vi "loadcontrsval.vi"(4 "error in":errorcluster, 5 "Array":refnum<vi>[](array[refnum]), 6 "Section":string, 7 "refnum in":T1) -> (0 "error out":errorcluster, 3 "refnum out":T1)   [LabVIEW 2010]
uses:
  <vilib>/Utility/config.llb/Config Data RefNum.ctl
  <vilib>/Utility/config.llb/Read Key (String).vi
  <vilib>/Utility/config.llb/Write Key (String).vi
  <vilib>/Utility/config.llb/Read Key (Path).vi
  <vilib>/Utility/config.llb/Write Key (Path).vi
  <vilib>/Utility/config.llb/Read Key (Double).vi
  <vilib>/Utility/config.llb/Write Key (Double).vi
  <vilib>/Utility/config.llb/Read Key (I32).vi
  <vilib>/Utility/config.llb/Write Key (I32).vi
  <vilib>/Utility/config.llb/Read Key (Boolean).vi
  <vilib>/Utility/config.llb/Write Key (Boolean).vi
  <vilib>/Utility/config.llb/NI_LVConfig.lvlib
panel:
  out "Array 2":string[](array[string])
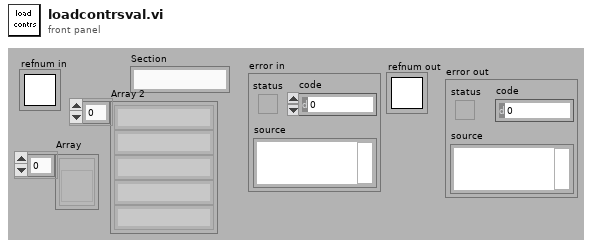
[diagram p1: front panel]
types:
  T1 = typedef "NI_LVConfig.lvlib/Config Data RefNum.ctl" = refnum<k1>
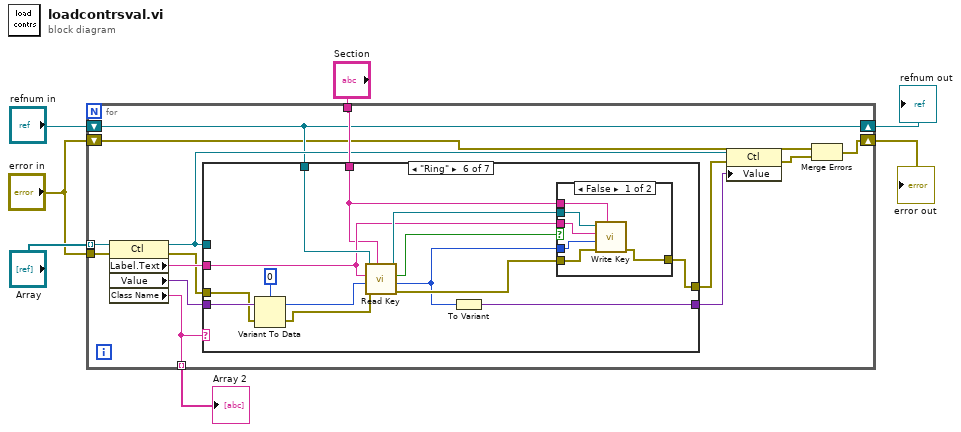
[diagram p0: block diagram]
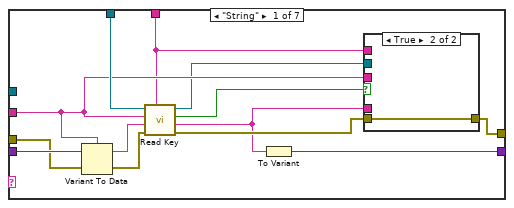
[diagram p2: hidden frame]
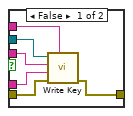
[diagram p3: hidden frame]
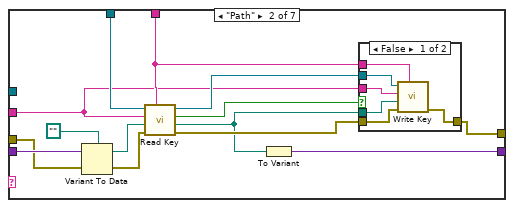
[diagram p4: hidden frame]
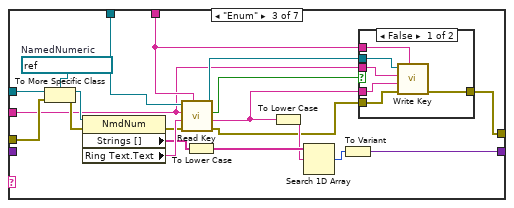
[diagram p6: hidden frame]
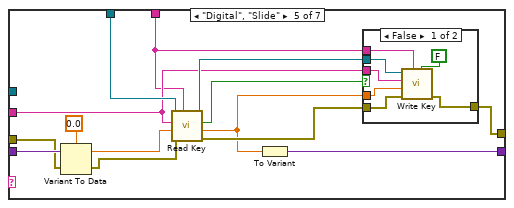
[diagram p9: hidden frame]
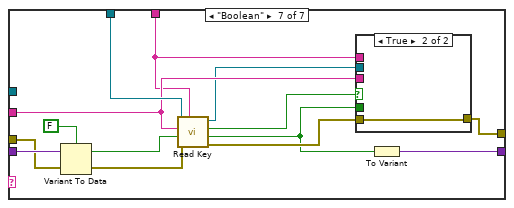
[diagram p12: hidden frame]
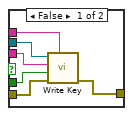
[diagram p13: hidden frame]
diagram:
  n1 = for {
    tunnel: "Section" -> [w18]
    tunnel: "Array" -> [w21] mode=indexing
    shift-right: [w14] -> w7
    shift-left: "refnum in" -> [w14]
    shift-right: [w9] -> w3
    shift-left: "error in" -> [w10]
    tunnel: [w20] -> w2 mode=indexing
    tunnel: "error in" -> [w11]
    n2 = property on="Property Node" class="Ctl"(reference=w21, error in=w11) -> (reference out=w15:refnum<vi>, error out=w13:errorcluster, "Label.Text"=w17:string, "Value"=w19:variant, "Class Name"=w20:string)
    n3 = case shown="\"Ring\"" w20 {
      tunnel: w19 -> [w34 w55 _ w91 w105 w127 w148]
      tunnel: w18 -> [w23 w45 w65 _ w93 w115 w135]
      tunnel: w14 -> [w32 w53 w79 _ w101 w123 w145]
      tunnel: w17 -> [w25 w44 w64 _ w94 w116 w139]
      tunnel: [w31 w52 w80 w91 w102 w124 w146] -> w16
      tunnel: w15 -> [_ _ w78 _ _ _ _]
      tunnel: w13 -> [w30 w50 w71 w90 w100 w122 w143]
      tunnel: [w22 w42 w67 w90 w92 w114 w138] -> w12
      frame "String" {
        n4 = Variant To Data(error in=w30, Variant=w34, type=w25) -> (error out=w29:errorcluster, data=w33:string)
        n5 = call-poly <vilib>:"Read Key.vi"("section"=w23, "error in (no error)"=w29, "default value"=w33, "key"=w25, "refnum"=w32) -> ("error out"=w27:errorcluster, "value"=w26:string, "found?"=w28:bool, "refnum out"=w24:T1)  [unwired: 3 in]
        n6 = To Variant(anything=w26) -> (Variant=w31:variant)
        n7 = case shown="True" w28 {
          tunnel: w27 -> [w40 w41]
          tunnel: [w39 w41] -> w22
          tunnel: w26 -> [w38 _]
          tunnel: w25 -> [w37 _]
          tunnel: w24 -> [w36 _]
          tunnel: w23 -> [w35 _]
          frame False {
            n8 = call-poly <vilib>:"Write Key.vi"("section"=w35, "error in (no error)"=w40, "value"=w38, "key"=w37, "refnum"=w36) -> ("error out"=w39:errorcluster)  [unwired: 4 in, 2 out]
          }
          frame True {
          }
        }
      }
      frame "Path" {
        n9 = Variant To Data(error in=w50, Variant=w55, type=path "") -> (error out=w49:errorcluster, data=w54:path)
        n10 = call-poly <vilib>:"Read Key.vi"("section"=w45, "error in (no error)"=w49, "default value"=w54, "key"=w44, "refnum"=w53) -> ("error out"=w47:errorcluster, "value"=w43:path, "found?"=w48:bool, "refnum out"=w46:T1)  [unwired: 3 in]
        n11 = To Variant(anything=w43) -> (Variant=w52:variant)
        n12 = case shown="False" w48 {
          tunnel: w47 -> [w61 w62]
          tunnel: w46 -> [w60 _]
          tunnel: w45 -> [w59 _]
          tunnel: w44 -> [w58 _]
          tunnel: w43 -> [w57 _]
          tunnel: [w56 w62] -> w42
          frame False {
            n13 = call-poly <vilib>:"Write Key.vi"("section"=w59, "error in (no error)"=w61, "value"=w57, "key"=w58, "refnum"=w60) -> ("error out"=w56:errorcluster)  [unwired: 4 in, 2 out]
          }
          frame True {
          }
        }
      }
      frame "Enum" {
        w82 = refnum<vi> refnum  # NamedNumeric
        n14 = To More Specific Class(target class=w82, reference=w78, error in=w71) -> (specific class reference=w81:refnum<vi>, error out=w70:errorcluster)
        n15 = property class="NmdNum"(reference=w81, error in=w70) -> (error out=w72:errorcluster, "Strings []"=w76:string[], "Ring Text.Text"=w77:string)  [unwired: 1 out]
        n16 = call-poly <vilib>:"Read Key.vi"("section"=w65, "error in (no error)"=w72, "default value"=w77, "key"=w64, "refnum"=w79) -> ("error out"=w68:errorcluster, "value"=w63:string, "found?"=w69:bool, "refnum out"=w66:T1)  [unwired: 3 in]
        n17 = To Lower Case(string=w76) -> (all lower case string=w75:string[])
        n18 = To Lower Case(string=w63) -> (all lower case string=w74:string)
        n19 = Search 1D Array(1D array=w75, element=w74) -> (index of element=w73:i32)  [unwired: 1 in]
        n20 = To Variant(anything=w73) -> (Variant=w80:variant)
        n21 = case shown="False" w69 {
          tunnel: w68 -> [w88 w89]
          tunnel: [w87 w89] -> w67
          tunnel: w66 -> [w86 _]
          tunnel: w65 -> [w85 _]
          tunnel: w64 -> [w84 _]
          tunnel: w63 -> [w83 _]
          frame False {
            n22 = call-poly <vilib>:"Write Key.vi"("section"=w85, "error in (no error)"=w88, "value"=w83, "key"=w84, "refnum"=w86) -> ("error out"=w87:errorcluster)  [unwired: 4 in, 2 out]
          }
          frame True {
          }
        }
      }
      frame "Any", Default {
      }
      frame "Digital", "Slide" {
        n23 = Variant To Data(error in=w100, Variant=w105, type=0.0 ("number")) -> (error out=w99:errorcluster, data=w103:dbl)
        n24 = call-poly <vilib>:"Read Key.vi"("section"=w93, "error in (no error)"=w99, "default value"=w103, "key"=w94, "refnum"=w101) -> ("error out"=w98:errorcluster, "value"=w97:dbl, "found?"=w95:bool, "refnum out"=w96:T1)  [unwired: 3 in]
        n25 = To Variant(anything=w97) -> (Variant=w102:variant)
        n26 = case shown="False" w95 {
          tunnel: w98 -> [w112 w113]
          tunnel: [w111 w113] -> w92
          tunnel: w97 -> [w110 _]
          tunnel: w96 -> [w109 _]
          tunnel: w94 -> [w108 _]
          tunnel: w93 -> [w106 _]
          frame False {
            n27 = call-poly <vilib>:"Write Key.vi"("use system decimal point (T)"=FALSE, "section"=w106, "error in (no error)"=w112, "value"=w110, "key"=w108, "refnum"=w109) -> ("error out"=w111:errorcluster)  [unwired: 3 in, 2 out]
          }
          frame True {
          }
        }
      }
      frame "Ring" {
        n28 = Variant To Data(error in=w122, Variant=w127, type=0 ("number")) -> (error out=w121:errorcluster, data=w125:i32)
        n29 = call-poly <vilib>:"Read Key.vi"("section"=w115, "error in (no error)"=w121, "default value"=w125, "key"=w116, "refnum"=w123) -> ("error out"=w120:errorcluster, "value"=w119:i32, "found?"=w117:bool, "refnum out"=w118:T1)  [unwired: 3 in]
        n30 = To Variant(anything=w119) -> (Variant=w124:variant)
        n31 = case shown="False" w117 {
          tunnel: w120 -> [w133 w134]
          tunnel: [w132 w134] -> w114
          tunnel: w119 -> [w131 _]
          tunnel: w118 -> [w130 _]
          tunnel: w116 -> [w129 _]
          tunnel: w115 -> [w128 _]
          frame False {
            n32 = call-poly <vilib>:"Write Key.vi"("section"=w128, "error in (no error)"=w133, "value"=w131, "key"=w129, "refnum"=w130) -> ("error out"=w132:errorcluster)  [unwired: 4 in, 2 out]
          }
          frame True {
          }
        }
      }
      frame "Boolean" {
        n33 = Variant To Data(error in=w143, Variant=w148, type=FALSE) -> (error out=w142:errorcluster, data=w147:bool)
        n34 = call-poly <vilib>:"Read Key.vi"("section"=w135, "error in (no error)"=w142, "default value"=w147, "key"=w139, "refnum"=w145) -> ("error out"=w141:errorcluster, "value"=w140:bool, "found?"=w137:bool, "refnum out"=w136:T1)  [unwired: 3 in]
        n35 = case shown="True" w137 {
          tunnel: w141 -> [w154 w155]
          tunnel: w140 -> [w153 _]
          tunnel: w139 -> [w152 _]
          tunnel: [w151 w155] -> w138
          tunnel: w136 -> [w150 _]
          tunnel: w135 -> [w149 _]
          frame False {
            n36 = call-poly <vilib>:"Write Key.vi"("section"=w149, "error in (no error)"=w154, "value"=w153, "key"=w152, "refnum"=w150) -> ("error out"=w151:errorcluster)  [unwired: 4 in, 2 out]
          }
          frame True {
          }
        }
        n37 = To Variant(anything=w140) -> (Variant=w146:variant)
      }
    }
    n38 = property class="Ctl"(reference=w15, error in=w12, "Value"=w16) -> (error out=w8:errorcluster)  [unwired: 1 out]
    n39 = Merge Errors(w10, w8) -> (w9:errorcluster)
  }
  "refnum out" <- w7
  "error out" <- w3
  "Array 2" <- w2
